vi "UI Set DisableState.vi"(7 "Enable?":bool=TRUE, 8 "error in (no error)":errorcluster, 11 "State Variables in":T1) -> (0 "error out":errorcluster, 3 "State Variables out":T1)   [LabVIEW 2019, in "Control Workspace Object.lvlib"]
uses:
  Control Workspace Object.lvlib
  Types/Workspace Object State Variables.ctl
  Types/UI.Refs.ctl
  Types/UDP Streaming Command Cluster.ctl
  Types/UDP Streaming State.ctl
  <vilib>/NI VeriStand/Display Template Support/DisplayTemplateSupport.llb/enum_Display Template Handler Minimal To Workspace.ctl
  Types/Workspace Object Cached Settings.ctl
  NationalInstruments.VeriStand.SystemStorage
  <vilib>/NI VeriStand/Execution/Workspace/WorkspaceAPI.ctl
  NationalInstruments.VeriStand.ClientAPI
  <vilib>/NI VeriStand/Display Template Support/DisplayTemplateSupport.llb/enum_Display Template Handler Minimal To Widget Msg.ctl
  <vilib>/NI VeriStand/Execution/Workspace/SystemStateRegEventRef.ctl
  <vilib>/NI VeriStand/Execution/Workspace/Target State Info.ctl
  <vilib>/NI VeriStand/Execution/Workspace/Target State.ctl
  <vilib>/NI VeriStand/Execution/Workspace/SystemStateEventRef.ctl
  <vilib>/NI VeriStand/Execution/Workspace/NI_VS Workspace ExecutionAPI.lvlib
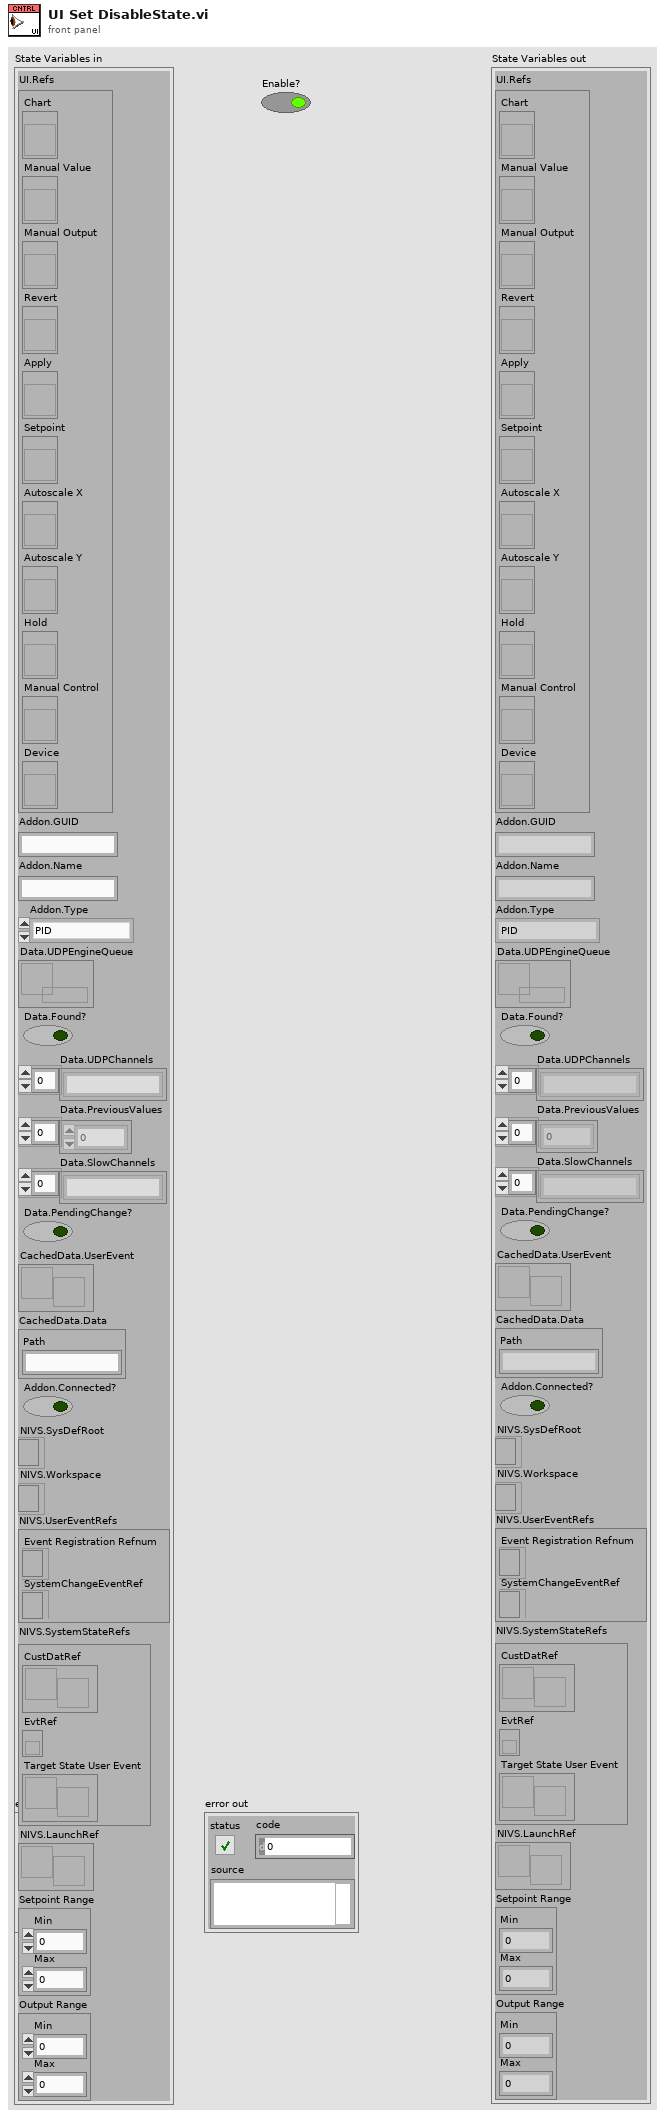
[diagram p1: front panel]
types:
  T1 = typedef "Control Workspace Object.lvlib/Workspace Object State Variables.ctl" = cluster{"UI.Refs":T2, "Addon.GUID":string, "Addon.Name":string, "Addon.Type":enum16{"PID", "Industrial"}, "Data.UDPEngineQueue":refnum<queue>, "Data.Found?":bool, "Data.UDPChannels":string[], "Data.PreviousValues":dbl[], "Data.SlowChannels":string[], "Data.PendingChange?":bool, "CachedData.UserEvent":refnum<user-event>, "CachedData.Data":T3, "Addon.Connected?":bool, "NIVS.SysDefRoot":refnum<k24>, "NIVS.Workspace":T4, "NIVS.UserEventRefs":cluster{"Event Registration Refnum":refnum<event-registration>, "SystemChangeEventRef":T5}, "NIVS.SystemStateRefs":T6, "NIVS.LaunchRef":refnum<user-event>, "Setpoint Range":cluster{"Min":dbl, "Max":dbl}, "Output Range":cluster{"Min":dbl, "Max":dbl}}
  T2 = typedef "Control Workspace Object.lvlib/UI.Refs.ctl" = cluster{"Chart":refnum<vi>, "Manual Value":refnum<vi>, "Manual Output":refnum<vi>, "Revert":refnum<vi>, "Apply":refnum<vi>, "Setpoint":refnum<vi>, "Autoscale X":refnum<vi>, "Autoscale Y":refnum<vi>, "Hold":refnum<vi>, "Manual Control":refnum<vi>, "Device":refnum<vi>}
  T3 = typedef "Control Workspace Object.lvlib/Workspace Object Cached Settings.ctl" = cluster{"Path":string}
  T4 = typedef "NI_VS Workspace ExecutionAPI.lvlib/WorkspaceAPI.ctl" = refnum<k24>
  T5 = typedef "NI_VS Workspace ExecutionAPI.lvlib/SystemStateRegEventRef.ctl" = refnum<event-registration>
  T6 = typedef "NI_VS Workspace ExecutionAPI.lvlib/SystemStateEventRef.ctl" = cluster{"CustDatRef":refnum<user-event>, "EvtRef":refnum<k27>, "Target State User Event":refnum<user-event>}
  T7 = enum8{"Enabled", "Disabled", "Disabled and Grayed Out"}
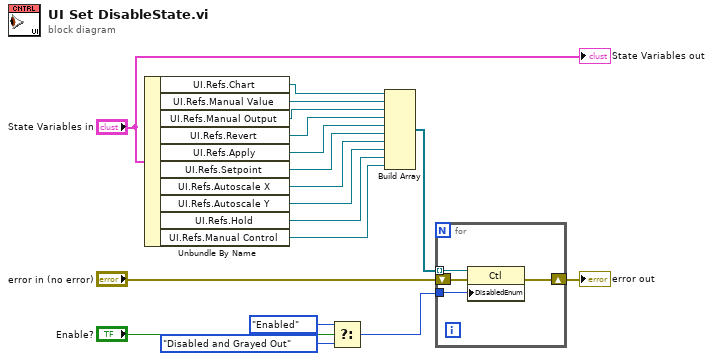
[diagram p0: block diagram]
diagram:
  n1 = Unbundle By Name("State Variables in") -> ("UI.Refs.Chart"=w18:refnum<vi>, "UI.Refs.Manual Value"=w17:refnum<vi>, "UI.Refs.Manual Output"=w16:refnum<vi>, "UI.Refs.Revert"=w15:refnum<vi>, "UI.Refs.Apply"=w14:refnum<vi>, "UI.Refs.Setpoint"=w13:refnum<vi>, "UI.Refs.Autoscale X"=w4:refnum<vi>, "UI.Refs.Autoscale Y"=w3:refnum<vi>, "UI.Refs.Hold"=w2:refnum<vi>, "UI.Refs.Manual Control"=w1:refnum<vi>)
  n2 = Select(t=T7."Enabled" ("Disabled"), s="Enable?", f=T7."Disabled and Grayed Out" ("Disabled")) -> (s? t:f=w5:T7)
  n3 = Build Array(w18, w17, w16, w15, w14, w13, w4, w3, w2, w1) -> (w12:refnum<vi>[])
  n4 = for {
    tunnel: w12 -> [w22] mode=indexing
    shift-right: [w20] -> w10
    shift-left: "error in (no error)" -> [w21]
    tunnel: w5 -> [w19]
    n5 = property class="Ctl"(reference=w22, error in=w21, "DisabledEnum"=w19) -> (error out=w20:errorcluster)  [unwired: 1 out]
  }
  "error out" <- w10
  "State Variables out" <- "State Variables in"
